vi "FPGA_Open.vi"(2 "error in":errorcluster) -> (0 "error out":errorcluster)   [LabVIEW 2009, in "FPGA.lvlib"]
doc: "Opens the FPGA reference and runs the FPGA code on the target. Needs to be called in the beginning of the program to be able to use FPGA_GetRef function and other implemented FPGA functionality."
uses:
  FPGA.lvlib
  <vilib>/rvi/interface/nirviOpenFPGA/nirviOpenFPGA.xnode
  FPGA Bitfiles/scmproject.lvproj_FPGA Target_RobotFPGA.vi.lvbitx
  RobotFPGA.vi
  <vilib>/FPGAPlugInAG/cRIO-9074/nirviIntfOpen_cRIO-9074.vi
  <vilib>/userDefined/High Color/nirio_resource_hc.ctl
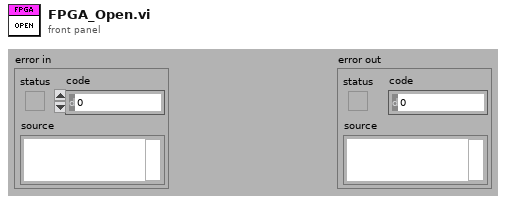
[diagram p1: front panel]
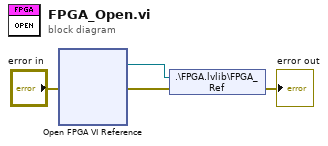
[diagram p0: block diagram]
diagram:
  n1 = xnode "Open FPGA VI Reference"("error in"="error in") -> ("FPGA VI Reference Out"=w4:refnum<k20>, "error out"=w3:errorcluster)  [unwired: 1 in]
  n2 = shared-variable ".\\FPGA.lvlib\\FPGA_Ref"(w4, error in=w3) -> (error out=→"error out":errorcluster)
